vi "Get Tag Value.vi"(5 "Litt/BigEnd":bool, 7 "DirEntries":T1[](array[typedef]), 8 "Tag Code":u16, 9 "Image Data in":u8[](array[numeric])) -> (0 "Array of Rationals":dbl[](array[numeric]), 1 "Multiple Values":u64[](array[numeric]), 2 "Single Value":u32, 3 "Image Data out":u8[](array[numeric]), 4 "Tag exists?":bool)   [LabVIEW 2015, in "Tiff reader.lvlib"]
doc: "Reads a single specific tag in the array of tags returned by Read Image File Directory.vi and returns the associated data (either a single value or multiple values). The definition and meaning of the various tags is given in the tiff specifications."
uses:
  Tiff reader.lvlib
  IFD Entry.ctl
  FieldTypes.ctl
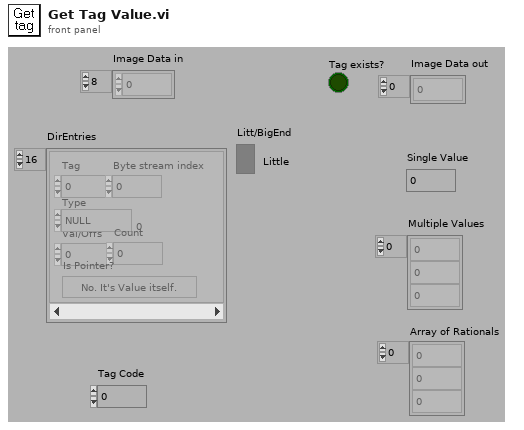
[diagram p1: front panel]
types:
  T1 = typedef "Tiff reader.lvlib/IFD Entry.ctl" = cluster{"Tag":u16, "Type":T2, "Count":u32, "Val/Offs":u32, "Is Pointer?":bool, "Byte stream index":i32}
  T2 = typedef "Tiff reader.lvlib/FieldTypes.ctl" = enum16{"NULL", "U8", "ASCII7", "U16", "U32", "RATIONAL", "SByte(I8)", "Undef(8Bit)", "I16", "I32", "SRat(4B:4B)", "SGL(4Byte)", "DBL(8Byte)"}
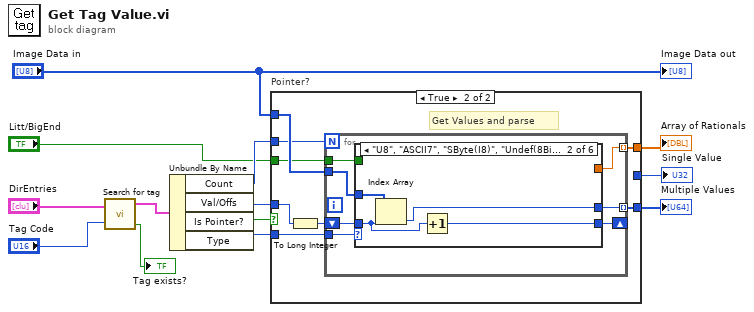
[diagram p0: block diagram]
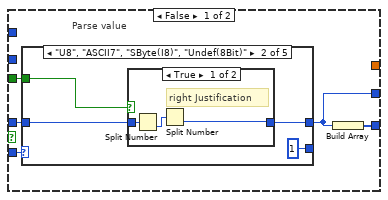
[diagram p2: hidden frame]
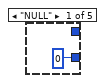
[diagram p3: hidden frame]
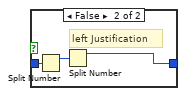
[diagram p4: hidden frame]
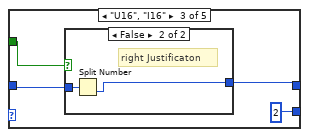
[diagram p5: hidden frame]
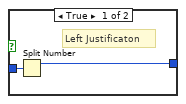
[diagram p6: hidden frame]
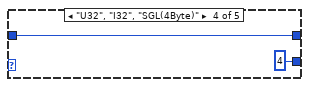
[diagram p7: hidden frame]
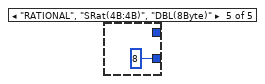
[diagram p8: hidden frame]
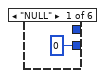
[diagram p9: hidden frame]
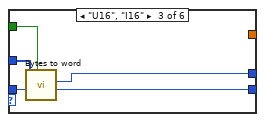
[diagram p10: hidden frame]
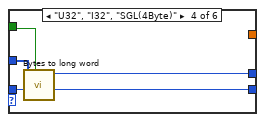
[diagram p11: hidden frame]
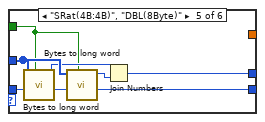
[diagram p12: hidden frame]
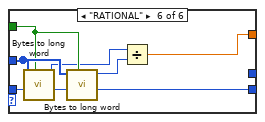
[diagram p13: hidden frame]
diagram:
  n1 = call "Search for tag.vi"("Directory"="DirEntries", "Tag"="Tag Code") -> ("Tag found"=w5:T1, "Tag exists?"=→"Tag exists?":bool)  [unwired: 1 out]
  n2 = Unbundle By Name(w5) -> ("Count"=w9:u32, "Val/Offs"=w12:u32, "Is Pointer?"=w13:bool, "Type"=w11:T2)
  n3 = case "Pointer?" shown="True" w13 {
    tunnel: w12 -> [w16 w46]
    tunnel: w11 -> [w17 w47]
    tunnel: "Image Data in" -> [_ w45]
    tunnel: [w18 w48] -> w10
    tunnel: w9 -> [_ w44]
    tunnel: [w15 _] -> w8
    tunnel: "Litt/BigEnd" -> [w14 w42]
    tunnel: [_ w41] -> w6
    frame False {
      # "Parse value"
      n4 = case shown="\"U8\", \"ASCII7\", \"SByte(I8)\", \"Undef(8Bit)\"" w17 {
        tunnel: [0 1 2 4 8] -> _
        tunnel: w16 -> [_ w22 w32 w38 _]
        tunnel: [_ w21 w31 w38 _] -> w15
        tunnel: w14 -> [_ w20 w30 _ _]
        frame "NULL" {
        }
        frame "U8", "ASCII7", "SByte(I8)", "Undef(8Bit)" {
          n5 = case shown="True" w20 {
            tunnel: w22 -> [w26 w29]
            tunnel: [w24 w27] -> w21
            frame True {
              # "right Justification"
              n6 = Split Number(x=w26) -> (lo(x)=w25:u16)  [unwired: 1 out]
              n7 = Split Number(x=w25) -> (lo(x)=w24:u8)  [unwired: 1 out]
            }
            frame False {
              # "left Justification"
              n8 = Split Number(x=w29) -> (hi(x)=w28:u16)  [unwired: 1 out]
              n9 = Split Number(x=w28) -> (hi(x)=w27:u8)  [unwired: 1 out]
            }
          }
        }
        frame "U16", "I16" {
          n10 = case shown="False" w30 {
            tunnel: w32 -> [w35 w37]
            tunnel: [w34 w36] -> w31
            frame True {
              # "Left Justificaton"
              n11 = Split Number(x=w35) -> (hi(x)=w34:u16)  [unwired: 1 out]
            }
            frame False {
              # "right Justificaton"
              n12 = Split Number(x=w37) -> (lo(x)=w36:u16)  [unwired: 1 out]
            }
          }
        }
        frame "U32", "I32", "SGL(4Byte)" {
        }
        frame "RATIONAL", "SRat(4B:4B)", "DBL(8Byte)" {
        }
      }
      n13 = Build Array(w15) -> (w18:u32[])
    }
    frame True {
      # "Get Values and parse"
      n14 = To Long Integer(number=w46) -> (32bit integer=w43:i32)
      n15 = for {
        N: w44 -> [_]
        tunnel: w45 -> [w54]
        tunnel: w47 -> [w55]
        tunnel: [w53] -> w48 mode=indexing
        shift-right: [w51] -> _
        shift-left: w43 -> [w52]
        tunnel: w42 -> [w50]
        tunnel: [w49] -> w41 mode=indexing
        n16 = case shown="\"U8\", \"ASCII7\", \"SByte(I8)\", \"Undef(8Bit)\"" w55 {
          tunnel: w54 -> [_ w60 w63 w70 w76 w84]
          tunnel: w52 -> [_ w58 w65 w69 w78 w86]
          tunnel: [_ w59 w62 w68 w73 _] -> w53
          tunnel: [0 ("Index+2") w57 w64 w67 w72 w83] -> w51
          tunnel: w50 -> [_ _ w61 w66 w71 w82]
          tunnel: [_ _ _ _ _ w79] -> w49
          frame "NULL" {
          }
          frame "U8", "ASCII7", "SByte(I8)", "Undef(8Bit)" {
            n17 = Index Array(array=w60, index=w58) -> (element=w59:u8)
            n18 = Increment(x=w58) -> (x+1=w57:i32)
          }
          frame "U16", "I16" {
            n19 = call "Bytes to word.vi"("Litt/BigEnd"=w61, "Index"=w65, "Image Data in"=w63) -> ("Index+2"=w64:i32, "Word"=w62:u16)  [unwired: 2 in, 3 out]
          }
          frame "U32", "I32", "SGL(4Byte)" {
            n20 = call "Bytes to long word.vi"("Litt/BigEnd"=w66, "Index"=w69, "Image Data in"=w70) -> ("Index+4"=w67:i32, "U32"=w68:u32)  [unwired: 5 out]
          }
          frame "SRat(4B:4B)", "DBL(8Byte)" {
            n21 = call "Bytes to long word.vi"("Litt/BigEnd"=w71, "Index"=w78, "Image Data in"=w76) -> ("Index+4"=w77:i32, "U32"=w75:u32)  [unwired: 5 out]
            n22 = call "Bytes to long word.vi"("Litt/BigEnd"=w71, "Index"=w77, "Image Data in"=w76) -> ("Index+4"=w72:i32, "U32"=w74:u32)  [unwired: 5 out]
            n23 = Join Numbers(hi=w75, lo=w74) -> ((hi.lo)=w73:u64)
          }
          frame "RATIONAL" {
            n24 = call "Bytes to long word.vi"("Litt/BigEnd"=w82, "Index"=w86, "Image Data in"=w84) -> ("Index+4"=w85:i32, "U32"=w81:u32)  [unwired: 5 out]
            n25 = call "Bytes to long word.vi"("Litt/BigEnd"=w82, "Index"=w85, "Image Data in"=w84) -> ("Index+4"=w83:i32, "U32"=w80:u32)  [unwired: 5 out]
            n26 = Divide(x=w81, y=w80) -> (x/y=w79:dbl)
          }
        }
      }
    }
  }
  "Multiple Values" <- w10
  "Single Value" <- w8
  "Array of Rationals" <- w6
  "Image Data out" <- "Image Data in"
